vi "All Child Values.vi"(11 "NewEntityTemplate in":refnum<class "Test1.lvclass">) -> (2 "All Values":refnum<class "Type.lvclass">[](array[class]))   [LabVIEW 2020, in "tests.lvlib" / "Test1.lvclass"]
uses:
  Test1.lvclass
  <vilib>/IlluminatedG/IG Conditum Base/Conditum/Columns/Type/Type.lvclass
  Test1.lvclass/Test1.ctl
  <vilib>/IlluminatedG/IG Conditum Base/Conditum/Columns/Integer/Integer.lvclass
  C:/Program Files (x86)/National Instruments/LabVIEW 2020/vi.lib/IlluminatedG/IG Conditum Base/Conditum/Columns/Type/Type.lvclass
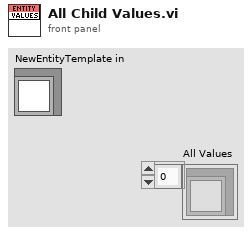
[diagram p1: front panel]
types:
  T1 = typedef "tests.lvlib/Test1.lvclass/Columns.ctl" = cluster{"<Placeholder>":refnum<class "Integer.lvclass">}
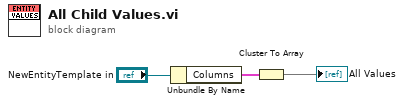
[diagram p0: block diagram]
diagram:
  n1 = Unbundle By Name("NewEntityTemplate in") -> ("Columns"=w2:T1)
  n2 = Cluster To Array(cluster=w2) -> (array=→"All Values":refnum<class "Integer.lvclass">[])
